vi "Connect.vi"(8 "error in":errorcluster, 11 "5105 in":refnum<class "5105.lvclass">) -> (0 "error out":errorcluster, 3 "5105 out":refnum<class "5105.lvclass">)   [LabVIEW 2019, in "5105.lvlib" / "5105.lvclass"]
uses:
  5105.lvclass
  C:/Users/Public/Documents/Development/builds/Instruments/Instruments.lvlibp/Library/Instruments.lvclass
  5105.lvclass/5105.ctl
  Accessors/Read Local Resource.vi
  builds/Instruments/Instruments.lvlibp/Accessors/Read Resource.vi
  builds/Instruments/Instruments.lvlibp/Accessors/Read Simulated.vi
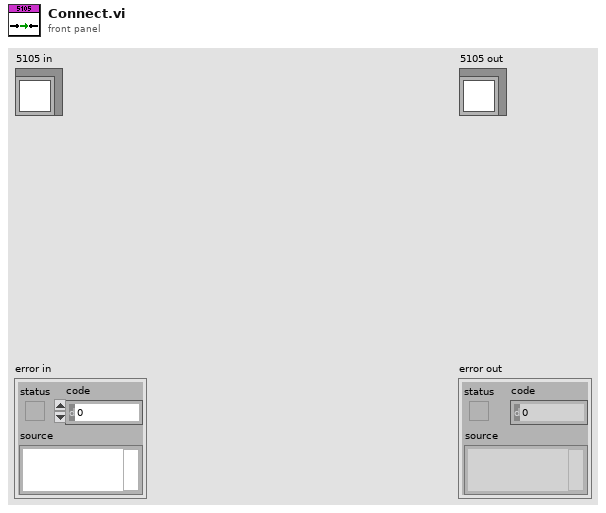
[diagram p1: front panel]
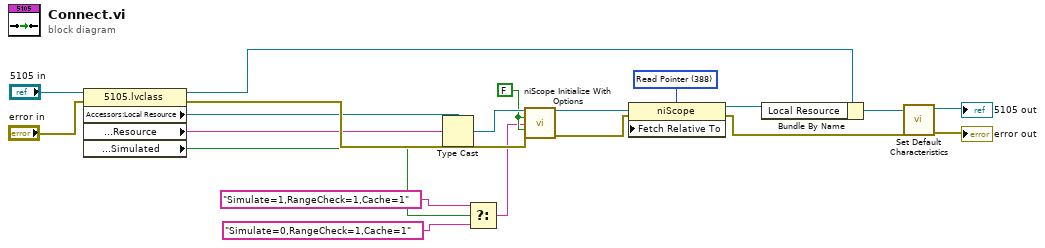
[diagram p0: block diagram]
diagram:
  w5 = 388 items=["Start"=482, "Trigger"=483, "Pretrigger"=477, "Now"=481, "Read Pointer"=388] ("Fetch:Fetch Relative To")
  w8 = FALSE
  n1 = property class="5105.lvclass"(reference="5105 in", error in="error in") -> (reference out=w16:refnum<class "5105.lvclass">, error out=w15:errorcluster, "Accessors:Local Resource"=w13:refnum<k15>, "Accessors:Configuration:Resource"=w14:string, "Accessors:Configuration:Simulated"=w12:bool)
  n2 = Type Cast(type=w13, x=w14) -> (*(type *) &x=w9:refnum<k15>)
  n3 = Select(t="Simulate=1,RangeCheck=1,Cache=1" ("option string"), s=w12, f="Simulate=0,RangeCheck=1,Cache=1" ("option string")) -> (s? t:f=w1:string)
  n4 = call <instrlib>:"niScope Initialize With Options.vi"("resource name"=w9, "id query"=w8, "option string"=w1, "reset device"=w8, "error in"=w15) -> ("instrument handle"=w7:refnum<k15>, "error out"=w4:errorcluster)  [unwired: 9 in]
  n5 = property class="niScope"(reference=w7, error in=w4, "Fetch Relative To"=w5) -> (reference out=w6:refnum<k15>, error out=w10:errorcluster)
  n6 = Bundle By Name(cluster=w16, "Local Resource"=w6) -> (w11:refnum<class "5105.lvclass">)
  n7 = call "Set Default Characteristics.vi"("error in (no error)"=w10, "5105 in"=w11) -> ("error out"=→"error out":errorcluster, "5105 out"=→"5105 out":refnum<class "5105.lvclass">)  [unwired: 8 in]
